vi "DiagramDisableStructure.vi"() -> ()   [LabVIEW 2019]
panel:
  out "Result":dbl
  in  "Numeric 2":dbl
  in  "Numeric":dbl
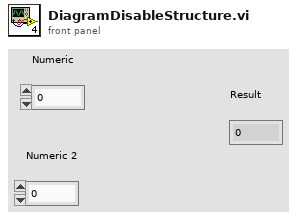
[diagram p1: front panel]
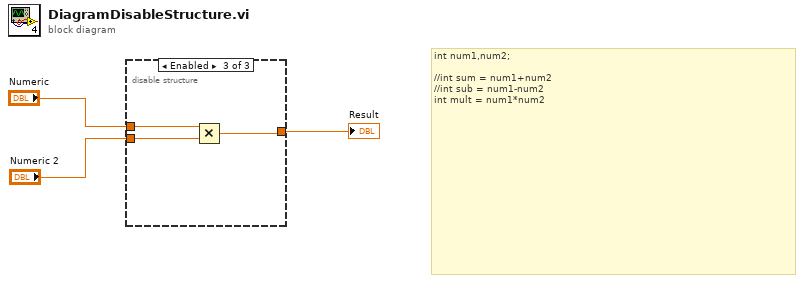
[diagram p0: block diagram]
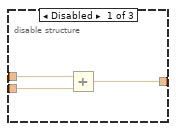
[diagram p2: hidden frame]
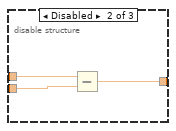
[diagram p3: hidden frame]
diagram:
  # "int num1,num2;\n\n//int sum = num1+num2\n//int sub = num1-num2\nint mult = num1*num2"
  n1 = disable-structure shown="Enabled" {
    disable-tunnel: "Numeric" -> [w6 w9 w12]
    disable-tunnel: "Numeric 2" -> [w5 w8 w11]
    disable-tunnel: [w4 w7 w10] -> w1
    frame Disabled {
      n2 = Add(x=w6, y=w5) -> (x+y=w4:dbl)
    }
    frame Disabled {
      n3 = Subtract(x=w9, y=w8) -> (x-y=w7:dbl)
    }
    frame Enabled {
      n4 = Multiply(x=w12, y=w11) -> (x*y=w10:dbl)
    }
  }
  "Result" <- w1
